vi "Query Voltage.vi"(8 "error in (no error)":errorcluster, 10 "Motor ID (0)":u8, 11 "VISA resource name":refnum<visa-resource-name>) -> (0 "error out":errorcluster, 2 "Voltage (V)":sgl, 3 "VISA resource name out":refnum<visa-resource-name>)   [LabVIEW 2016, in "Dynamixel Motor.lvlib"]
doc: "Gets the motor's voltage."
uses:
  Dynamixel Motor.lvlib
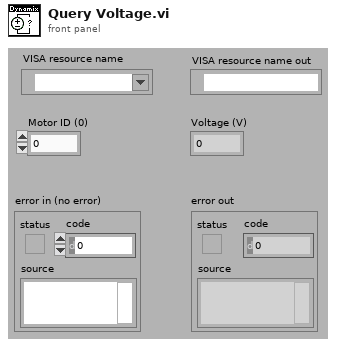
[diagram p1: front panel]
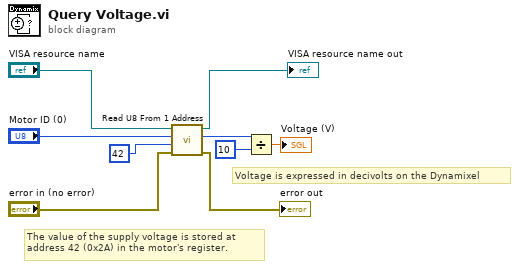
[diagram p0: block diagram]
diagram:
  # "The value of the supply voltage is stored at \naddress 42 (0x2A) in the motor's register."
  # "Voltage is expressed in decivolts on the Dynamixel"
  n1 = call "Read U8 From 1 Address.vi"("Error in (no error)"="error in (no error)", "Address number (0)"=u8 42 ("Address # DEC"), "Motor ID (0)"="Motor ID (0)", "VISA resource name"="VISA resource name") -> ("error out"=→"error out":errorcluster, "Data"=w5:u8, "VISA resource name out"=→"VISA resource name out":refnum<visa-resource-name>)  [unwired: 5 in]
  n2 = Divide(x=w5, y=u8 10) -> (x/y=→"Voltage (V)":dbl)
